vi "Corazon.vi"(10 "Paso":dbl, 11 "Tiempo":dbl) -> (2 "Array 2":dbl[](array[numeric]), 3 "Array":dbl[](array[numeric]))   [LabVIEW 2011]
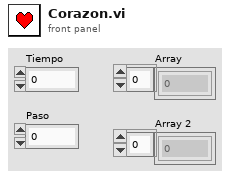
[diagram p1: front panel]
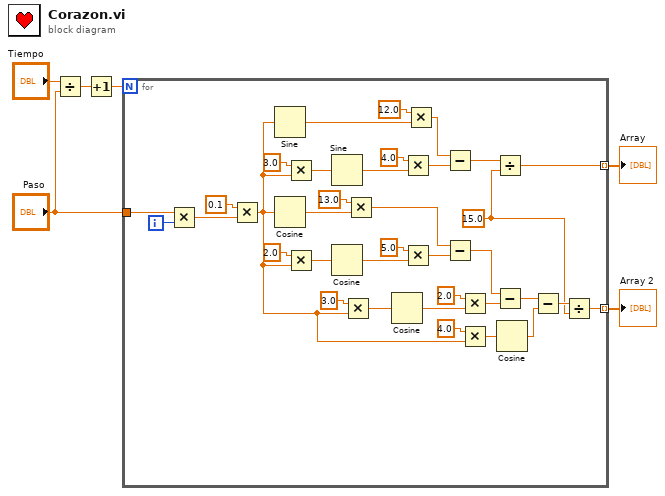
[diagram p0: block diagram]
diagram:
  n1 = Divide(x="Tiempo", y="Paso") -> (x/y=w5:dbl)
  n2 = Increment(x=w5) -> (x+1=w4:dbl)
  n3 = for {
    N: w4 -> [_]
    tunnel: [w30] -> w3 mode=indexing
    tunnel: [w9] -> w2 mode=indexing
    tunnel: "Paso" -> [w7]
    i -> [w42]
    w8 = 15.0 ("y")
    n4 = Multiply(x=w7, y=w42) -> (x*y=w41:dbl)
    n5 = Multiply(x=0.1, y=w41) -> (x*y=w23:dbl)
    n6 = Sine(x=w23) -> (sin(x)=w38:dbl)
    n7 = Cosine(x=w23) -> (cos(x)=w22:dbl)
    n8 = Multiply(x=3.0, y=w23) -> (x*y=w32:dbl)
    n9 = Multiply(x=2.0, y=w23) -> (x*y=w29:dbl)
    n10 = Sine(x=w32) -> (sin(x)=w39:dbl)
    n11 = Cosine(x=w29) -> (cos(x)=w21:dbl)
    n12 = Multiply(x=3.0, y=w23) -> (x*y=w28:dbl)
    n13 = Multiply(x=13.0, y=w22) -> (x*y=w16:dbl)
    n14 = Cosine(x=w28) -> (cos(x)=w20:dbl)
    n15 = Multiply(x=4.0, y=w39) -> (x*y=w34:dbl)
    n16 = Multiply(x=5.0, y=w21) -> (x*y=w15:dbl)
    n17 = Multiply(x=12.0, y=w38) -> (x*y=w33:dbl)
    n18 = Subtract(x=w33, y=w34) -> (x-y=w35:dbl)
    n19 = Subtract(x=w16, y=w15) -> (x-y=w14:dbl)
    n20 = Multiply(x=2.0, y=w20) -> (x*y=w13:dbl)
    n21 = Multiply(x=4.0, y=w23) -> (x*y=w27:dbl)
    n22 = Divide(x=w35, y=w8) -> (x/y=w30:dbl)
    n23 = Subtract(x=w14, y=w13) -> (x-y=w11:dbl)
    n24 = Cosine(x=w27) -> (cos(x)=w12:dbl)
    n25 = Subtract(x=w11, y=w12) -> (x-y=w10:dbl)
    n26 = Divide(x=w10, y=w8) -> (x/y=w9:dbl)
  }
  "Array" <- w3
  "Array 2" <- w2
